vi "Swap_Gate.vi"(6 "Top Gate?":bool, 8 "error in (no error)":errorcluster, 9 "d CtrlLine in":refnum<class "CtrlLine.lvclass">, 10 "u CtrlLine in":refnum<class "CtrlLine.lvclass">, 11 "QuWire in":refnum<class "QuWire.lvclass">) -> (0 "error out":errorcluster, 1 "d CtrlLine out":refnum<class "CtrlLine.lvclass">, 3 "QuWire out":refnum<class "QuWire.lvclass">)   [LabVIEW 2020, in "QuWire.lvclass"]
uses:
  QuWire.lvclass
  CtrlLine/CtrlLine.lvclass
  QuWire.lvclass/QuWire.ctl
  SimAlg/PrllPerElement/PrllPerElmnt.lvclass
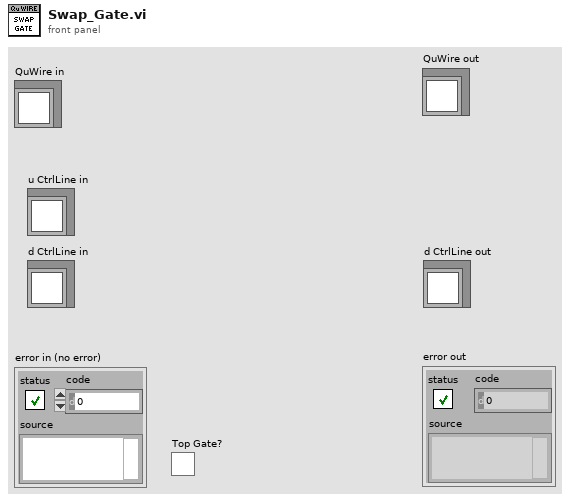
[diagram p1: front panel]
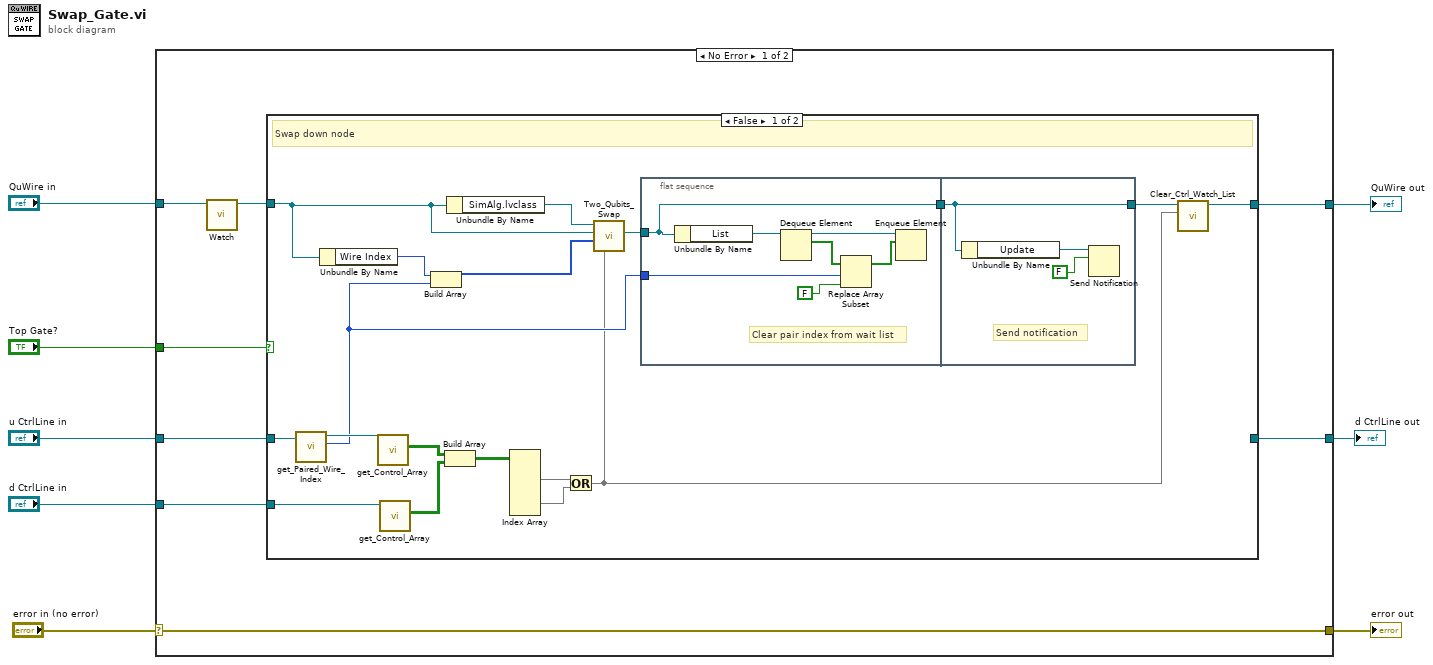
[diagram p0: block diagram]
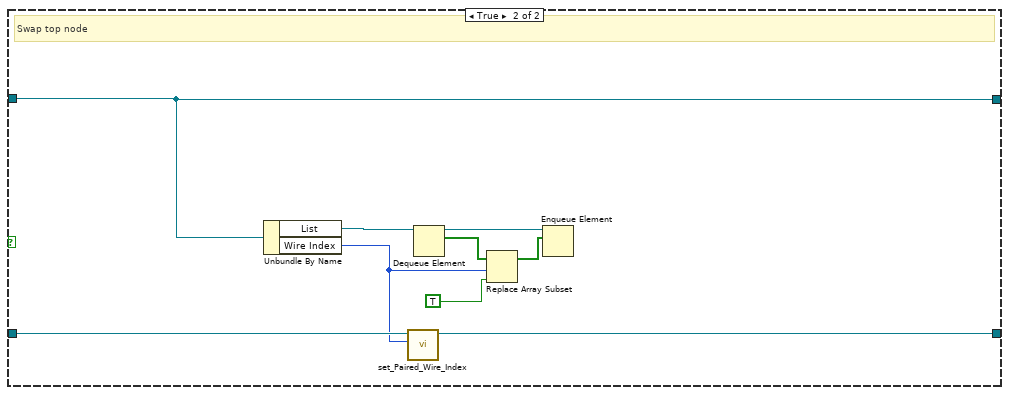
[diagram p2: hidden frame]
diagram:
  n1 = case shown="No Error" "error in (no error)" {
    selector: "error in (no error)" -> [w16 w56]
    tunnel: [w16 w56] -> w7
    tunnel: [w13 w55] -> w5
    tunnel: "QuWire in" -> [w14 w55]
    tunnel: "u CtrlLine in" -> [w15 w54]
    tunnel: "d CtrlLine in" -> [w12 _]
    tunnel: "Top Gate?" -> [w11 _]
    tunnel: [w10 w54] -> w1
    frame No Error {
      n2 = call "Watch.vi"("QuWire in"=w14) -> ("QuWire out"=w9:refnum<class "QuWire.lvclass">)  [unwired: 9 in, 1 out]
      n3 = case shown="False" w11 {
        tunnel: w15 -> [w26 w46]
        tunnel: w9 -> [w27 w48]
        tunnel: [w18 w48] -> w13
        tunnel: w12 -> [w33 _]
        tunnel: [_ w47] -> w10
        frame False {
          # "Swap down node"
          n4 = call "get_Paired_Wire_Index.vi"("CtrlLine in"=w26) -> ("Paired Wire Index"=w22:i32, "CtrlLine out"=w25:refnum<class "CtrlLine.lvclass">)  [unwired: 8 in, 1 out]
          n5 = Unbundle By Name(w27) -> ("Wire Index"=w24:i32)
          n6 = call "get_Control_Array.vi"("CtrlLine in"=w25) -> ("Control Array"=w29:bool[][])  [unwired: 8 in, 2 out]
          n7 = call "get_Control_Array.vi"("CtrlLine in"=w33) -> ("Control Array"=w28:bool[][])  [unwired: 8 in, 2 out]
          n8 = Build Array(w24, w22) -> (w23:i32[])
          n9 = Build Array(w29, w28) -> (w30:bool[][][])
          n10 = Unbundle By Name(w27) -> ("SimAlg.lvclass"=w34:refnum<class "PrllPerElmnt.lvclass">)
          n11 = Index Array(array=w30) -> (element #1=w31:bool[][], element #2=w32:bool[][])  [unwired: 6 in]
          n12 = Or(x=w31, y=w32) -> (x .or. y?=w20:bool[][])
          n13 = call-dynamic "Two_Qubits_Swap.vi"("ControlArray"=w20, "SwapingWiresIndex"=w23, "QuWire in"=w27, "SimAlg in"=w34) -> ("QuWire out"=w21:refnum<class "QuWire.lvclass">)  [unwired: 5 in, 2 out]
          n14 = flat-sequence {
            tunnel: w22 -> [w36]
            tunnel: w21 -> [w35]
            tunnel: [w35] -> w17
            tunnel: [w44] -> w19
            tunnel: w17 -> [w44]
            frame #0 {
              # "Clear pair index from wait list"
              n15 = Unbundle By Name(w35) -> ("List"=w41:refnum<queue>)
              n16 = Dequeue Element(queue=w41) -> (queue out=w40:refnum<queue>, element=w39:bool[])  [unwired: 2 in, 2 out]
              n17 = Replace Array Subset(array=w39, new element=FALSE ("new element/subarray"), index=w36) -> (w38:bool[])
              n18 = Enqueue Element(queue=w40, element=w38) -> ()  [unwired: 2 in, 3 out]
            }
            frame #1 {
              # "Send notification"
              n19 = Unbundle By Name(w44) -> ("Update"=w42:refnum<notifier>)
              n20 = Send Notification(notification=FALSE, notifier=w42) -> ()  [unwired: 1 in, 2 out]
            }
          }
          n21 = call "Clear_Ctrl_Watch_List.vi"("Control Array"=w20, "QuWire in"=w19) -> ("QuWire out"=w18:refnum<class "QuWire.lvclass">)  [unwired: 9 in]
        }
        frame True {
          # "Swap top node"
          n22 = Unbundle By Name(w48) -> ("List"=w53:refnum<queue>, "Wire Index"=w45:i32)
          n23 = call "set_Paired_Wire_Index.vi"("Paired Wire Index"=w45, "CtrlLine in"=w46) -> ("CtrlLine out"=w47:refnum<class "CtrlLine.lvclass">)  [unwired: 8 in, 1 out]
          n24 = Dequeue Element(queue=w53) -> (queue out=w52:refnum<queue>, element=w51:bool[])  [unwired: 2 in, 2 out]
          n25 = Replace Array Subset(array=w51, new element=TRUE ("new element/subarray"), index=w45) -> (w49:bool[])
          n26 = Enqueue Element(queue=w52, element=w49) -> ()  [unwired: 2 in, 3 out]
        }
      }
    }
    frame Error {
    }
  }
  "error out" <- w7
  "QuWire out" <- w5
  "d CtrlLine out" <- w1
